vi "GetCurrentOS.vi"() -> (2 "Betriebssystem:Name":string)   [LabVIEW 2017, in "libpqutility.lvlib"]
doc: "return OS at runtime"
uses:
  libpqutility.lvlib
panel:
  out "Betriebssystem:Version":string
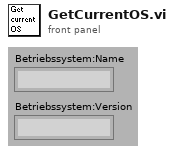
[diagram p1: front panel]
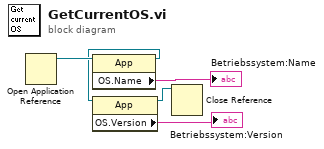
[diagram p0: block diagram]
diagram:
  n1 = Open Application Reference() -> (3:w3:refnum<vi>)  [unwired: 4 in, 1 out]
  n2 = property class="App"(reference=w3) -> (reference out=w2:refnum<vi>, "OS.Name"=→"Betriebssystem:Name":string)  [unwired: 1 in, 1 out]
  n3 = property class="App"(reference=w2) -> (reference out=w1:refnum<vi>, "OS.Version"=→"Betriebssystem:Version":string)  [unwired: 1 in, 1 out]
  n4 = Close Reference(reference=w1) -> ()  [unwired: 1 in, 1 out]
